vi "ReadXML3.vi"(7 "ParamsUI":T2 {"Rectangle"."Rotation" format="%.2f"; "Rectangle"."Left" scale=0.0..1024.0; "Rectangle"."Right" scale=0.0..1024.0}, 10 "Name":string="A1", 11 "基路径":path) -> (3 "ParamsUI 2":T2 {"Rectangle"."Rotation" format="%.2f"; "Rectangle"."Left" scale=0.0..1024.0; "Rectangle"."Right" scale=0.0..1024.0})   [LabVIEW 2015]
uses:
  <vilib>/Utility/xml.llb/Read From XML File(string).vi
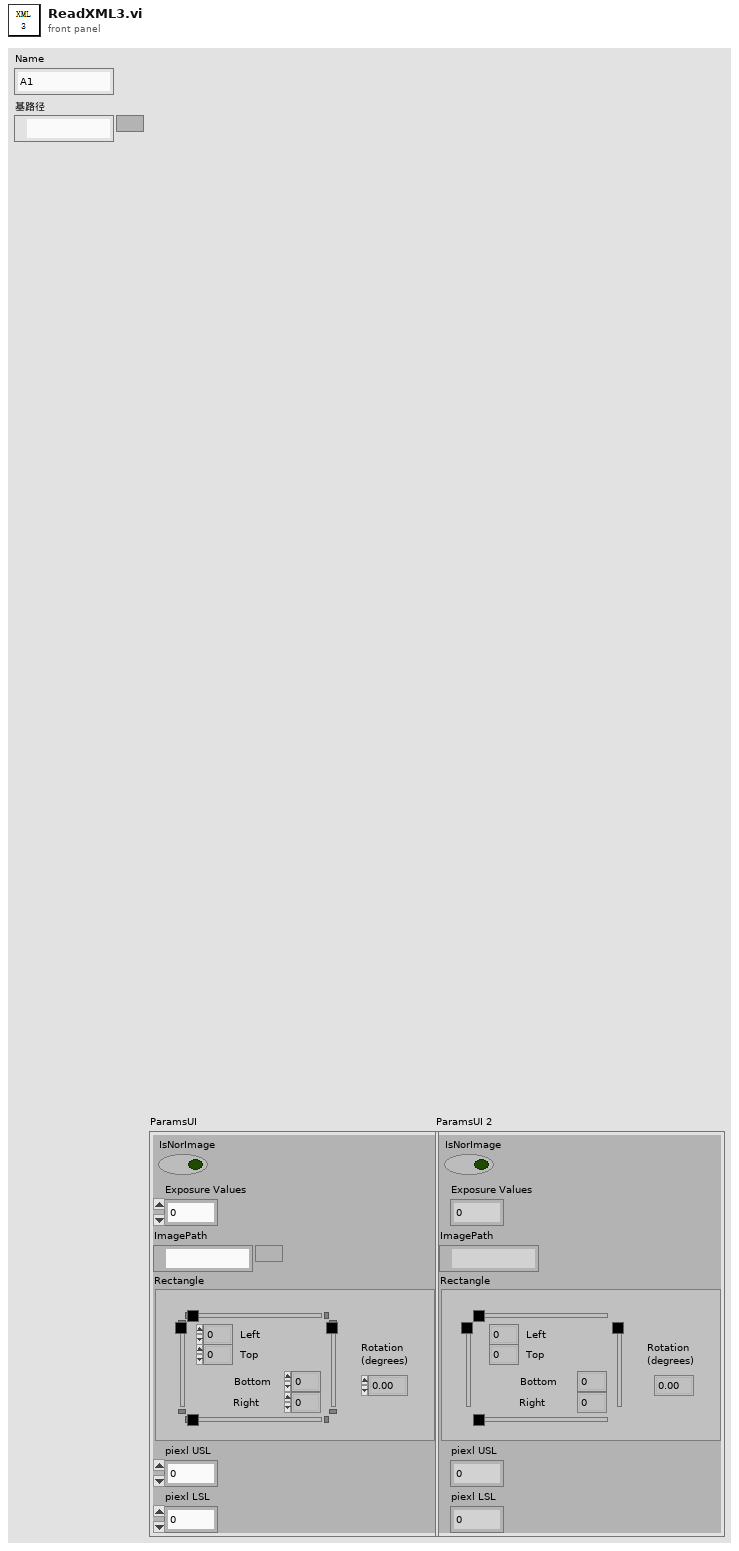
[diagram p1: front panel]
types:
  T1 = typedef "IMAQ Rectangle" = cluster{"Left":i32, "Top":i32, "Right":i32, "Bottom":i32, "Rotation":dbl}
  T2 = cluster{"IsNorImage":bool, "Exposure Values":u32, "ImagePath":path, "Rectangle":T1, "piexl USL":dbl, "piexl LSL":dbl}
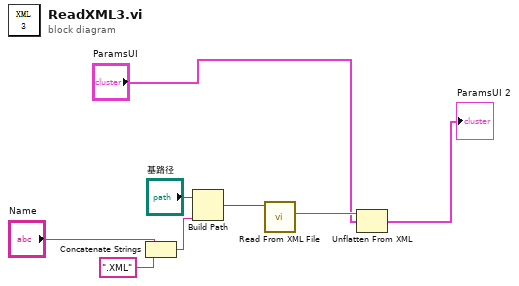
[diagram p0: block diagram]
diagram:
  n1 = Concatenate Strings("Name", ".XML" ("字符串")) -> (w4:string)
  n2 = Build Path(base path="基路径", name or relative path=w4) -> (appended path=w8:path)
  n3 = call-poly <vilib>:"Read From XML File.vi"("XML File Path"=w8) -> ("XML Elements"=w7:string)  [unwired: 8 in, 2 out]
  n4 = Unflatten From XML(xml string=w7, type="ParamsUI") -> (value=→"ParamsUI 2":T2)  [unwired: 1 in, 1 out]
